vi "Counter with Race Condition.vi"() -> ()   [LabVIEW 2012]
panel:
  out "运行总数":i32
  in  "停止按钮":bool
  out "循环计数差":i32
  out "循环计数2":i32
  out "循环计数1":i32
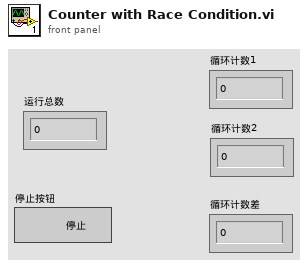
[diagram p1: front panel]
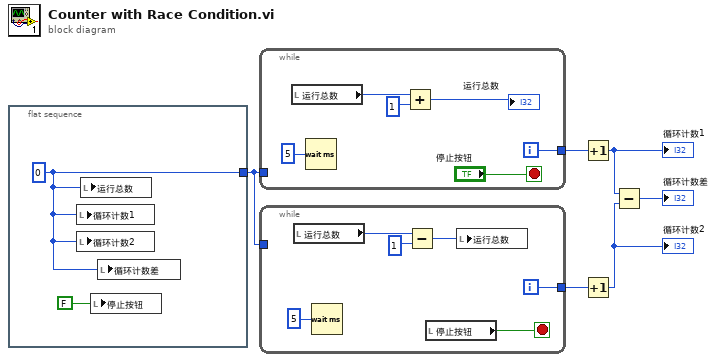
[diagram p0: block diagram]
diagram:
  n1 = flat-sequence {
    tunnel: [w7] -> w4
    frame #0 {
      w7 = 0 ("运行总数")
      n2 = local write "循环计数1"(w7) -> ()
      n3 = local write "循环计数2"(w7) -> ()
      n4 = local write "运行总数"(w7) -> ()
      n5 = local write "停止按钮"(FALSE ("停止按钮")) -> ()
      n6 = local write "循环计数差"(w7) -> ()
    }
  }
  n7 = while {
    tunnel: [w10] -> w6
    tunnel: w4 -> [_]
    i -> [w10]
    stop <- "停止按钮" stop-if-true
    n8 = local read "运行总数"() -> (w11:i32)
    n9 = Wait (ms) ("等待(ms)")(milliseconds to wait=u32 5 ("等待时间（毫秒）")) -> ()  [unwired: 1 out]
    n10 = Add ("加")(x=w11, y=1 ("x")) -> (x+y=→"运行总数":i32)
  }
  n11 = while {
    tunnel: [w18] -> w5
    tunnel: w4 -> [_]
    i -> [w18]
    stop <- w20 stop-if-true
    n12 = local read "运行总数"() -> (w17:i32)
    n13 = Wait (ms) ("等待(ms)")(milliseconds to wait=u32 5 ("等待时间（毫秒）")) -> ()  [unwired: 1 out]
    n14 = Subtract ("减")(x=w17, y=1 ("x")) -> (x-y=w15:i32)
    n15 = local read "停止按钮"() -> (w20:bool)
    n16 = local write "运行总数"(w15) -> ()
  }
  n17 = Increment ("加1")(x=w6) -> (x+1=w3:i32)
  "循环计数1" <- w3
  n18 = Increment ("加1")(x=w5) -> (x+1=w2:i32)
  "循环计数2" <- w2
  n19 = Subtract ("减")(x=w3, y=w2) -> (x-y=→"循环计数差":i32)
